vi "Read U32 Var.vi"(2 "错误输入（无错误）":errorcluster, 3 "Tag IN":string, 4 "Ds PLCTags IN":T1[](array[typedef])) -> (0 "error out":errorcluster, 1 "U32 Var out":dbl)   [LabVIEW 2014]
uses:
  DataSocket_Tags.ctl
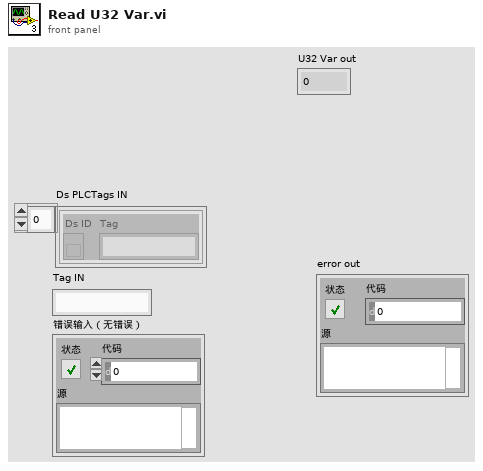
[diagram p1: front panel]
types:
  T1 = typedef "DataSocket_Tags.ctl" = cluster{"Ds ID":refnum<k13>, "Tag":string}
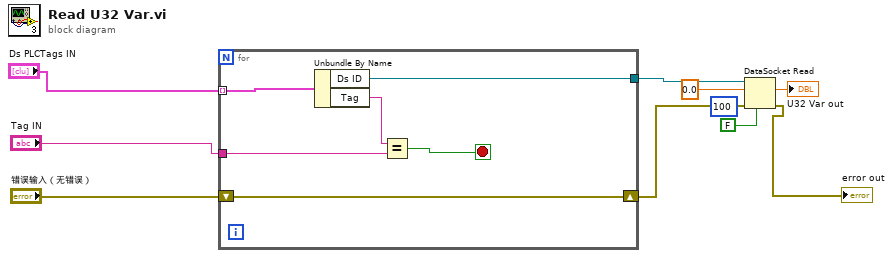
[diagram p0: block diagram]
diagram:
  n1 = for {
    tunnel: "Ds PLCTags IN" -> [w16] mode=indexing
    tunnel: "Tag IN" -> [w14]
    tunnel: [w12] -> w6
    shift-right: [w11] -> w5
    shift-left: "错误输入（无错误）" -> [w11]
    stop <- w13 stop-if-true
    n2 = Unbundle By Name(w16) -> ("Ds ID"=w12:refnum<k13>, "Tag"=w15:string)
    n3 = Equal?(x=w15, y=w14) -> (x = y?=w13:bool)
  }
  n4 = DataSocket Read(6:FALSE ("等待更新值(T)"), 8:w5, 9:100 ("毫秒超时(10000)"), 10:0.0, 11:w6) -> (0:→"error out":errorcluster, 2:→"U32 Var out":dbl)  [unwired: 5 out]
